vi "FM.vi"() -> ()   [LabVIEW 2018]
uses:
  <vilib>/Analysis/8numeric.llb/1D Numeric Integration.vi
  <vilib>/measure/maspectr.llb/FFT Power Spectrum and PSD for 1 Chan.vi
  <vilib>/Analysis/NI_AALPro.lvlib
  <vilib>/measure/NI_MAPro.lvlib
panel:
  out "FM":dbl[](graph)
  out "FM PS":cluster{"f0":dbl, "df":dbl, "magnitude":dbl[]}(graph)
  out "Modulador  Graph":dbl[](graph)
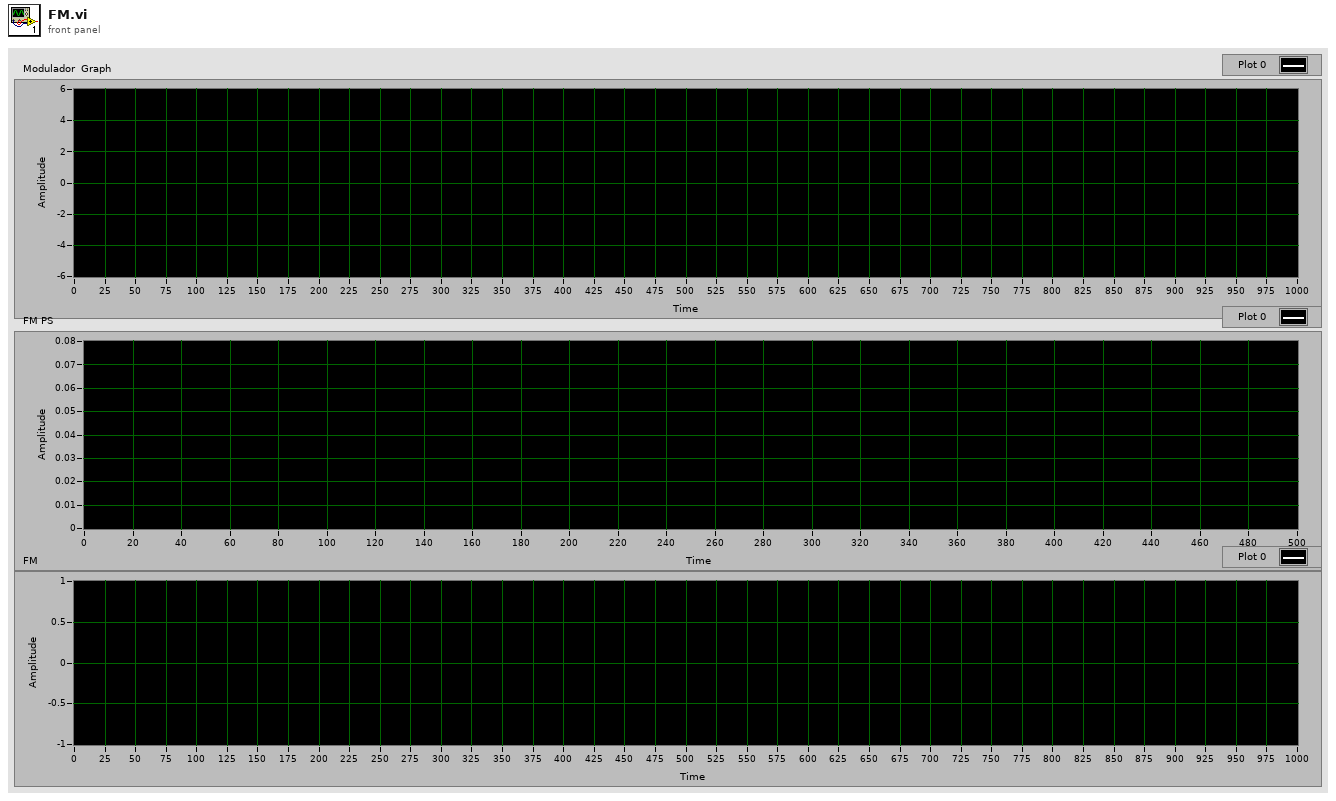
[diagram p1: front panel]
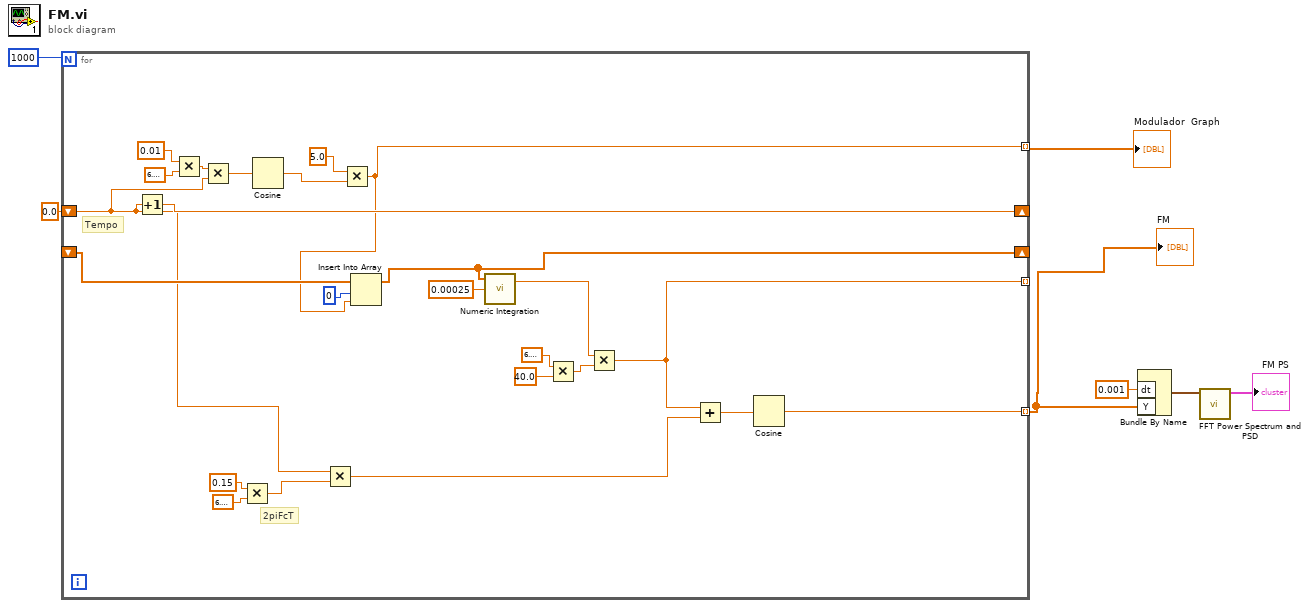
[diagram p0: block diagram]
diagram:
  n1 = for {
    N: 1000 -> [_]
    shift-right: [w24] -> _
    shift-left: _ -> [w26]
    tunnel: [w8] -> _ mode=indexing
    tunnel: [w11] -> w5 mode=indexing
    shift-right: [w23] -> _
    shift-left: 0.0 -> [w9]
    tunnel: [w21] -> w3 mode=indexing
    # "2piFcT"
    # "Tempo"
    n2 = Increment(x=w9) -> (x+1=w23:dbl)
    n3 = Multiply(x=0.01, y=6.283185307179586) -> (x*y=w30:dbl)
    n4 = Multiply(x=w30, y=w9) -> (x*y=w29:dbl)
    n5 = Multiply(x=0.15, y=6.283185307179586) -> (x*y=w22:dbl)
    n6 = Cosine(x=w29) -> (cos(x)=w31:dbl)
    n7 = Multiply(x=w9, y=w22) -> (x*y=w13:dbl)
    n8 = Multiply(x=5.0 ("y"), y=w31) -> (x*y=w11:dbl)
    n9 = Insert Into Array(array=w26, index=0, new element=w11) -> (w24:dbl[])
    n10 = call-poly <vilib>:"Numeric Integration.vi"("dt"=0.00025, "Input Array"=w24) -> ("result"=w17:dbl)  [unwired: 1 in, 1 out]
    n11 = Multiply(x=6.283185307179586, y=40.0) -> (x*y=w18:dbl)
    n12 = Multiply(x=w17, y=w18) -> (x*y=w8:dbl)
    n13 = Add(x=w8, y=w13) -> (x+y=w14:dbl)
    n14 = Cosine(x=w14) -> (cos(x)=w21:dbl)
  }
  "Modulador  Graph" <- w5
  "FM" <- w3
  n15 = Bundle By Name("dt"=0.001, "Y"=w3) -> (w4:waveform(dbl))  [unwired: 1 in]
  n16 = call-poly <vilib>:"FFT Power Spectrum and PSD.vi"("time signal"=w4) -> ("Power Spectrum / PSD"=→"FM PS":cluster{"f0":dbl, "df":dbl, "magnitude":dbl[]})  [unwired: 7 in, 3 out]
